vi "GetText.vi"(8 "error in":errorcluster, 11 "group in":refnum<class "group node.lvclass">) -> (0 "error out":errorcluster, 1 "additional text":string, 2 "text":string, 3 "group out":refnum<class "group node.lvclass">, 4 "glyph":string)   [LabVIEW 2013, in "group node.lvclass"]
uses:
  group node.lvclass
  group node.lvclass/group node.ctl
  Configuration Framework/serializable configuration/read metadata property.vi
  group configuration/group configuration.lvclass
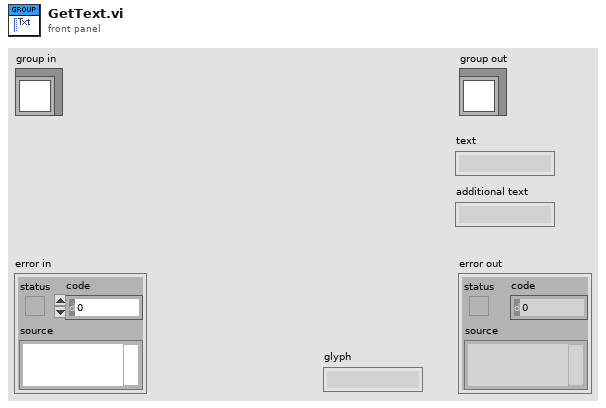
[diagram p1: front panel]
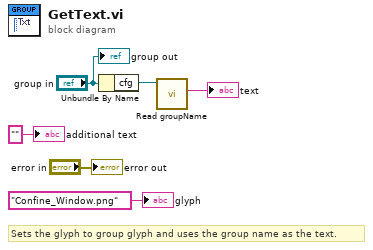
[diagram p0: block diagram]
diagram:
  # "Sets the glyph to group glyph and uses the group name as the text."
  n1 = Unbundle By Name("group in") -> ("cfg"=w2:refnum<class "group configuration.lvclass">)
  n2 = call "Read groupName.vi"("group configuration in"=w2) -> ("groupName"=→"text":string)  [unwired: 8 in, 2 out]
  "error out" <- "error in"
  "group out" <- "group in"
  "additional text" <- "" ("additional text")
  "glyph" <- "Confine_Window.png" ("glyph")
